vi "Day 4 Puzzle 2.vi"(11 "Path":path) -> ()   [LabVIEW 2021]
uses:
  <vilib>/Utility/file.llb/Read Delimited Spreadsheet (string).vi
panel:
  out "Number of contained":i32
  out "Overlap":bool[](array[boolean])
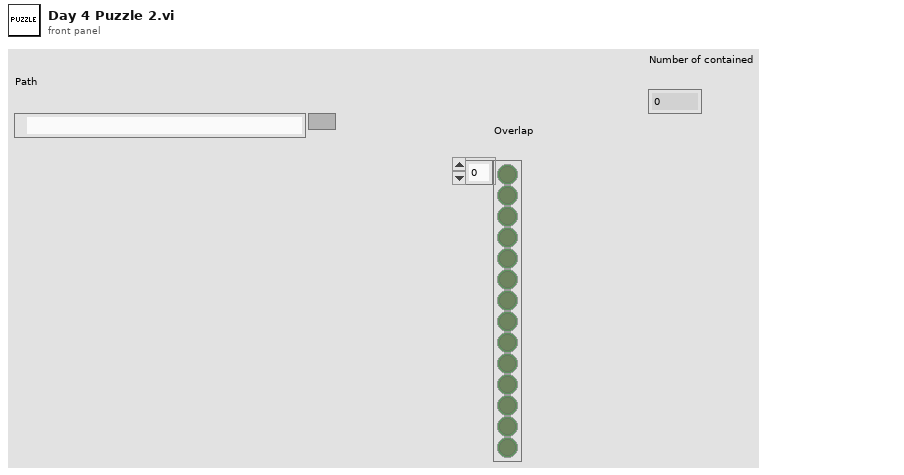
[diagram p1: front panel]
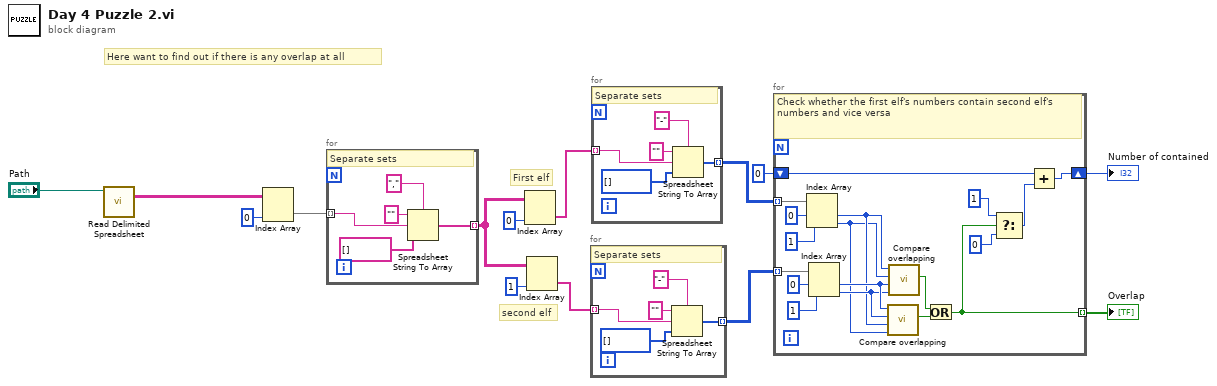
[diagram p0: block diagram]
diagram:
  # "Here want to find out if there is any overlap at all"
  # "second elf"
  # "First elf"
  n1 = call-poly <vilib>:"Read Delimited Spreadsheet.vi"("file path (dialog if empty)"="Path") -> ("all rows"=w13:string[][])  [unwired: 9 in, 5 out]
  n2 = Index Array(array=w13, index (col)=0 ("disabled index (col)")) -> (element=w11:string[])  [unwired: 1 in]
  n3 = for {
    tunnel: w11 -> [w17] mode=indexing
    tunnel: [w15] -> w8 mode=indexing
    # "Separate sets"
    n4 = Spreadsheet String To Array(delimiter (Tab)=",", format string="", spreadsheet string=w17, array type (2D Dbl)=string[] []) -> (array=w15:string[])
  }
  n5 = Index Array(array=w8, index (col)=0 ("disabled index (col)")) -> (element=w7:string[])  [unwired: 1 in]
  n6 = Index Array(array=w8, index (col)=1 ("disabled index (col)")) -> (element=w6:string[])  [unwired: 1 in]
  n7 = for {
    tunnel: w6 -> [w23] mode=indexing
    tunnel: [w21] -> w4 mode=indexing
    # "Separate sets"
    n8 = Spreadsheet String To Array(delimiter (Tab)="-", format string="", spreadsheet string=w23, array type (2D Dbl)=i32[] []) -> (array=w21:i32[])
  }
  n9 = for {
    tunnel: w7 -> [w28] mode=indexing
    tunnel: [w26] -> w5 mode=indexing
    # "Separate sets"
    n10 = Spreadsheet String To Array(delimiter (Tab)="-", format string="", spreadsheet string=w28, array type (2D Dbl)=i32[] []) -> (array=w26:i32[])
  }
  n11 = for {
    tunnel: w5 -> [w47] mode=indexing
    tunnel: w4 -> [w42] mode=indexing
    tunnel: [w30] -> w3 mode=indexing
    shift-right: [w39] -> w2
    shift-left: 0 -> [w41]
    # "Check whether the first elf's numbers contain second elf's numbers and vice versa"
    n12 = Index Array(array=w47, index #1=0 ("index"), index #2=1 ("index")) -> (element #1=w34:i32, element #2=w33:i32)
    n13 = Index Array(array=w42, index #1=0 ("index"), index #2=1 ("index")) -> (element #1=w36:i32, element #2=w35:i32)
    n14 = call "Compare overlapping.vi"("8"=w33, "6"=w34, "4"=w35, "2"=w36) -> ("Boolean"=w31:bool)  [unwired: 7 in]
    n15 = call "Compare overlapping.vi"("8"=w35, "6"=w36, "4"=w33, "2"=w34) -> ("Boolean"=w32:bool)  [unwired: 7 in]
    n16 = Or(x=w32, y=w31) -> (x .or. y?=w30:bool)
    n17 = Select(t=1, s=w30, f=0) -> (s? t:f=w40:i32)
    n18 = Add(x=w41, y=w40) -> (x+y=w39:i32)
  }
  "Overlap" <- w3
  "Number of contained" <- w2
